vi "curvefit_usingmodel.vi"(4 "Y":dbl[](array[numeric]), 5 "initial parameters":dbl[](array[numeric]), 6 "Run Number":dbl, 7 "param upper bounds":dbl[](array[numeric]), 8 "Weight":dbl[](array[numeric]), 9 "X":dbl[](array[numeric]), 10 "param lower bounds":dbl[](array[numeric]), 11 "model":refnum<vi>) -> (0 "where error string":string, 1 "Variances":dbl[](array[numeric]), 2 "Fitted Curve":dbl[](array[numeric]), 3 "best fit parameters":dbl[](array[numeric]))   [LabVIEW 2022 SP3]
uses:
  <vilib>/gmath/NumericalOptimization/Nonlinear Curve Fit LM bound.vi
  <vilib>/Analysis/Matrix/Numeric/Conversions/Matrix To Array - RM.vi
  <vilib>/Analysis/Matrix/NI_Matrix.lvlib
  <vilib>/gmath/NI_Gmath.lvlib
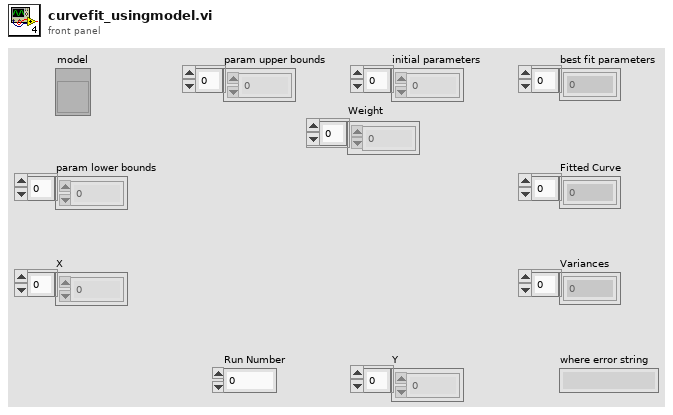
[diagram p1: front panel]
types:
  T1 = cluster{"param upper bounds":dbl[], "param lower bounds":dbl[]}
  T2 = typedef "NI_Matrix.lvlib/RealMatrix.ctl" = dbl[][]
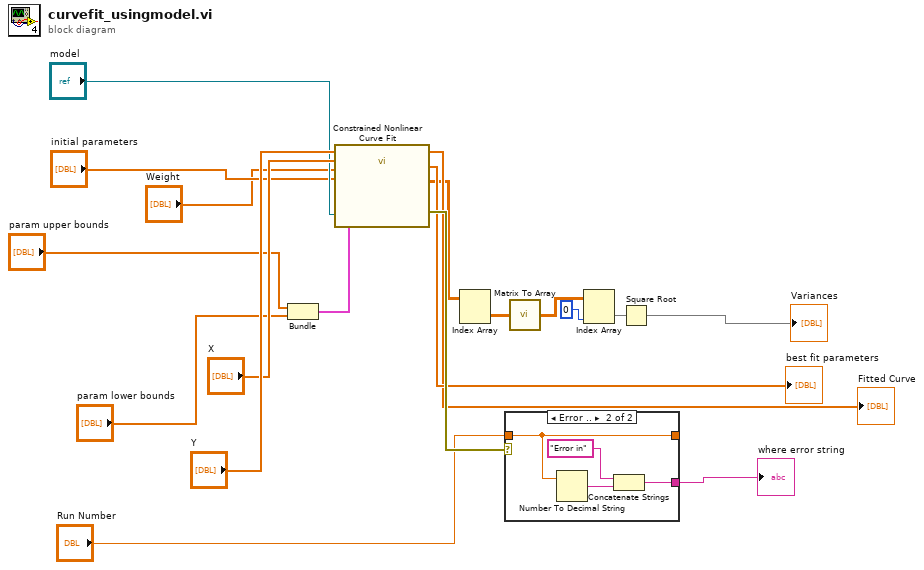
[diagram p0: block diagram]
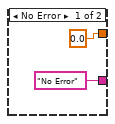
[diagram p2: hidden frame]
diagram:
  n1 = Bundle("param upper bounds"="param upper bounds", "param lower bounds"="param lower bounds") -> (w13:T1)  [unwired: 1 in]
  n2 = call-poly <vilib>:"Constrained Nonlinear Curve Fit.vi"("Y"="Y", "f(x,a)"="model", "X"="X", "Weight"="Weight", "initial parameters"="initial parameters", "parameter bounds"=w13) -> ("best nonlinear fit"=→"Fitted Curve":dbl[], "best fit parameters"=→"best fit parameters":dbl[], "covariance"=w2:T2, "error out"=w18:errorcluster)  [unwired: 4 in, 2 out]
  n3 = Index Array(array=w2) -> (element=w3:T2)  [unwired: 2 in]
  n4 = case shown="Error .." w18 {
    tunnel: ["No Error" ("group name in") w25] -> w19
    tunnel: "Run Number" -> [_ w22]
    tunnel: [0.0 w22] -> _
    frame No Error {
    }
    frame Error {
      n5 = Number To Decimal String(number=w22) -> (decimal integer string=w24:string)  [unwired: 1 in]
      n6 = Concatenate Strings("Error in" ("group name in"), w24) -> (w25:string)
    }
  }
  "where error string" <- w19
  n7 = call-poly <vilib>:"Matrix To Array.vi"("Real Matrix"=w3) -> ("Real 2D Array"=w4:dbl[][])
  n8 = Index Array(array=w4, index (col)=0 ("disabled index (col)")) -> (element=w6:dbl[])  [unwired: 1 in]
  n9 = Square Root ("Square Root.vi")(x=w6) -> (sqrt(x)=→"Variances":dbl[])
